vi "DimostratoreTest.vi"() -> ()   [LabVIEW 2019]
doc: "Dimostratore API\n\nFunzionamento:\n1. Seleziona postazione e data\n Conferma\n Ottieni un array con tutti i test della postazione selezionata in base alla data\n2. Seleziona quale test eseguire\n Conferma che tutti gli assets dei test sono disponibili\n Mostra tutti gli step di un test\n3. Seleziona Step da eseguire inserendo anche un valore di prova\n Il risultato dello step viene riprodotto nell'outcome\n\nFunzionamento alternativo\n1. Imposta uno Step Id e conferma\n2. Inserisci un valore di prova e ottieni l'outcome"
uses:
  ByteGSAPIBase.lvclass
  TypeDef/MachineStates.ctl
  TypeDef/Test.ctl
  TypeDef/Asset.ctl
  TypeDef/Step.ctl
  <vilib>/Utility/miscctls.llb/LVStringsAndValuesArrayTypeDef_I32.ctl
panel:
  in  "Exit":bool=TRUE
  out "Step Name":string
  in  "Home":bool
  in  "Indietro":bool
  out "Infos":string
  in  "Duration":dbl
  in  "Ottieni Passaggio Step":bool
  in  "Step Id":i32
  in  "Valore Prova":dbl
  in  "Inizia Step":bool
  in  "Seleziona Step":i32(ring) items=["Plug and set the Power Supply"=36]
  in  "Inizia Test":bool
  in  "Seleziona Test":i32(ring)
  out "error out":errorcluster
  in  "error in (no error)":errorcluster
  in  "Ottieni Test Per Postazione":bool
  in  "ByteGSAPIBase in":refnum<class "ByteGSAPIBase.lvclass">
  in  "Data Partenza":timestamp format="%<%x>T"
  in  "Postazione":enum16{"POST 1", "POST 2"}(ring)
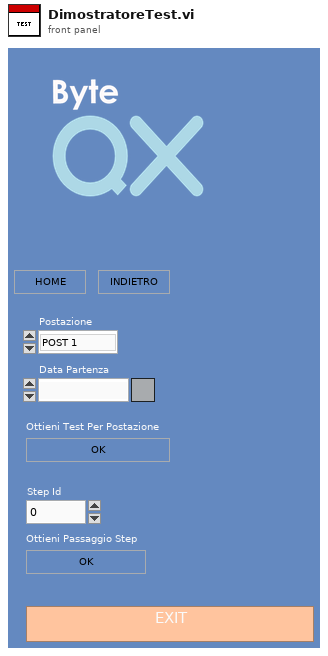
[diagram p1: front panel]
types:
  T1 = typedef "ByteGSWebAPI.lvlib/ByteGSAPIBase.lvclass/Step.ctl" = cluster{"id":i32, "descrizione":string, "prova":string, "assets":T2[], "criterio_accettazione":string, "valore_criterio_accettazione_max":dbl, "valore_criterio_accettazione_min":dbl, "udm_criterio_accettazione":string, "duration_prova":string, "udm_duration_prova":string, "valore_prova":dbl, "outcome":string, "ordine":i32, "user":i32, "link_automation":string, "instruction_automation":string, "data_completamento_checklist":timestamp}
  T2 = typedef "ByteGSWebAPI.lvlib/ByteGSAPIBase.lvclass/Asset.ctl" = cluster{"descrizione":string, "slug":string, "id":i32}
  T3 = typedef "ByteGSWebAPI.lvlib/ByteGSAPIBase.lvclass/Test.ctl" = cluster{"titolo":string, "descrizione":string, "statoprova":string, "assets":T2[], "id":i32, "data_apertura_prova":timestamp}
  T4 = typedef "MachineStates.ctl" = enum16{"Initialize", "Idle", "GetLimsTestsForBench", "AssetsCheck", "GetLimsTestSteps", "UpdateLimsTestStep", "GetLimsTestStep", "Indietro", "UpdateLimsTestStepAutomation"}
  T5 = cluster{"Postazione":refnum<vi>, "Data Partenza":refnum<vi>, "Ottieni Test Per Postazione":refnum<vi>, "Step Id":refnum<vi>, "Ottieni Passaggio Step":refnum<vi>, "Seleziona Test":refnum<vi>, "Inizia Test":refnum<vi>, "Seleziona Step":refnum<vi>, "Valore Prova":refnum<vi>, "Inizia Step":refnum<vi>, "Infos":refnum<vi>, "Duration":refnum<vi>, "Step Name":refnum<vi>, "Exit":refnum<vi>}
  T6 = cluster{"ByteGSAPIBase in":refnum<class "ByteGSAPIBase.lvclass">, "Array dei Test":T3[], "Steps Array":T1[]}
  T7 = typedef "LVStringsAndValuesArrayTypeDef_I32.ctl" = cluster{"String":string, "Value":i32}[]
  T8 = cluster{"Postazione":enum16{"POST 1", "POST 2"}, "Data Partenza":timestamp, "Seleziona Test":i32, "Seleziona Step":i32, "Valore Prova":dbl, "Step Id":i32, "Duration":dbl}
  T9 = cluster{"Postazione":enum16{"POST 1", "POST 2"}, "Data Partenza":timestamp}
  T10 = typedef "UpdateLimsTestStepData.ctl" = cluster{"duration_prova":string, "udm_duration_prova":string, "valore_prova":dbl, "outcome":string, "data_completamento_checklist":timestamp, "link_automation":string, "instruction_automation":string}
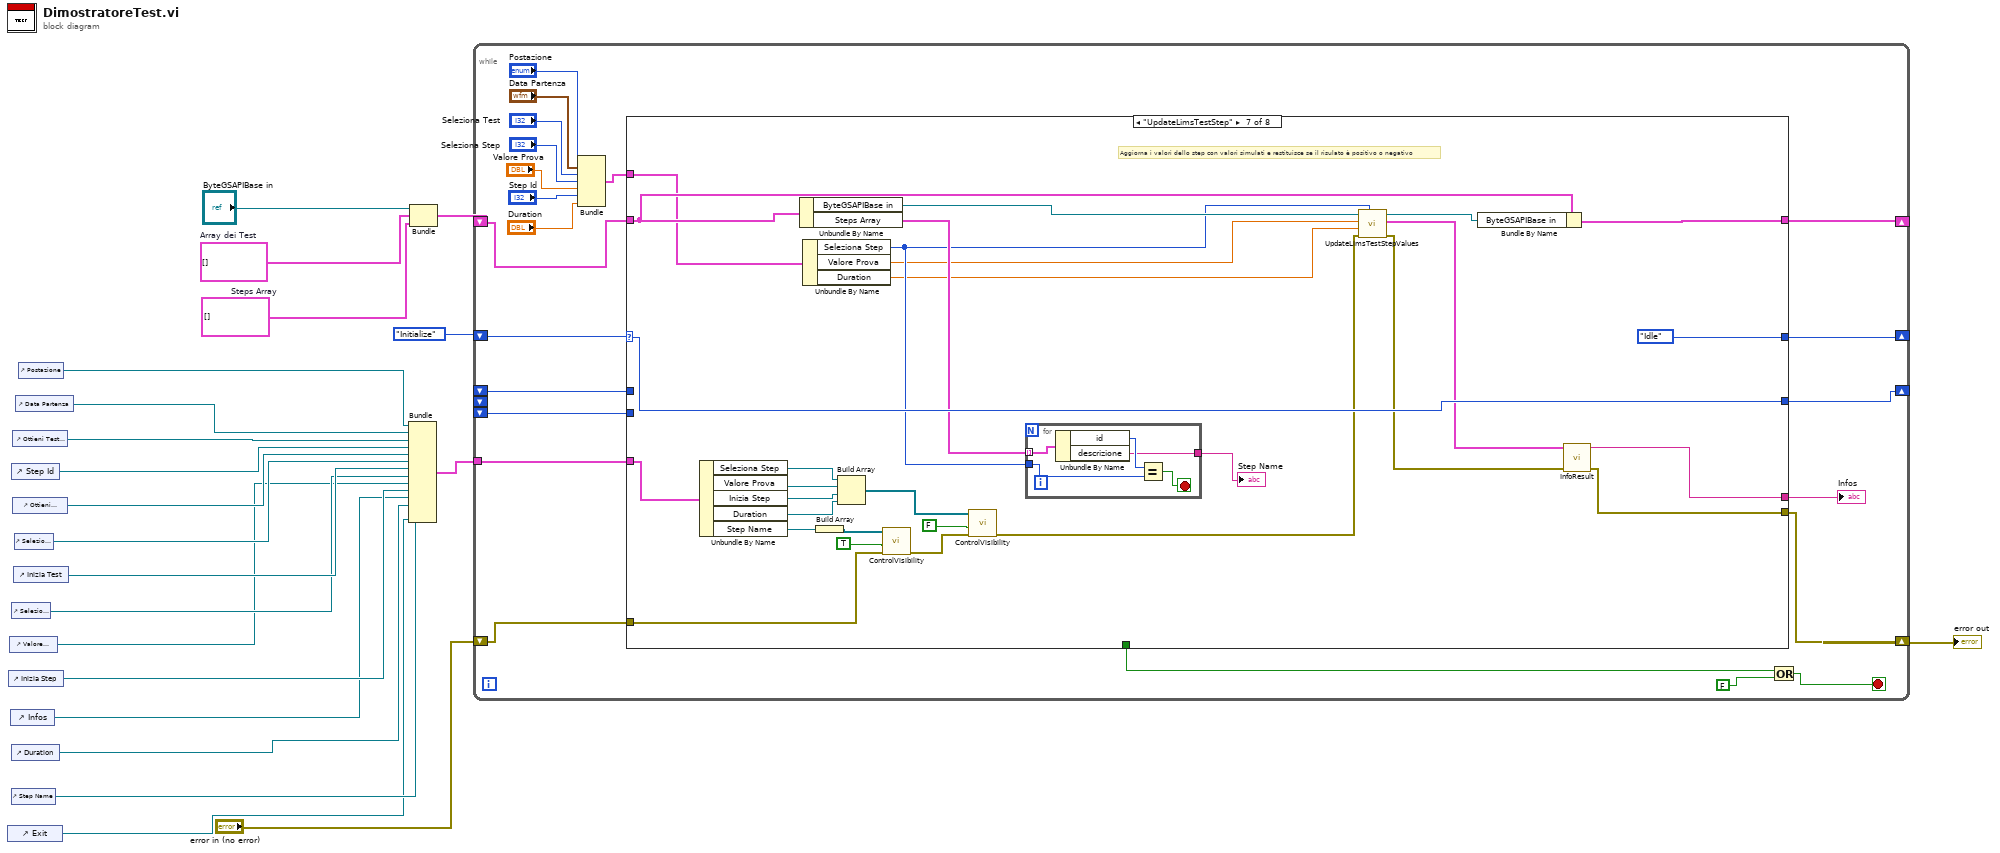
[diagram p0: block diagram]
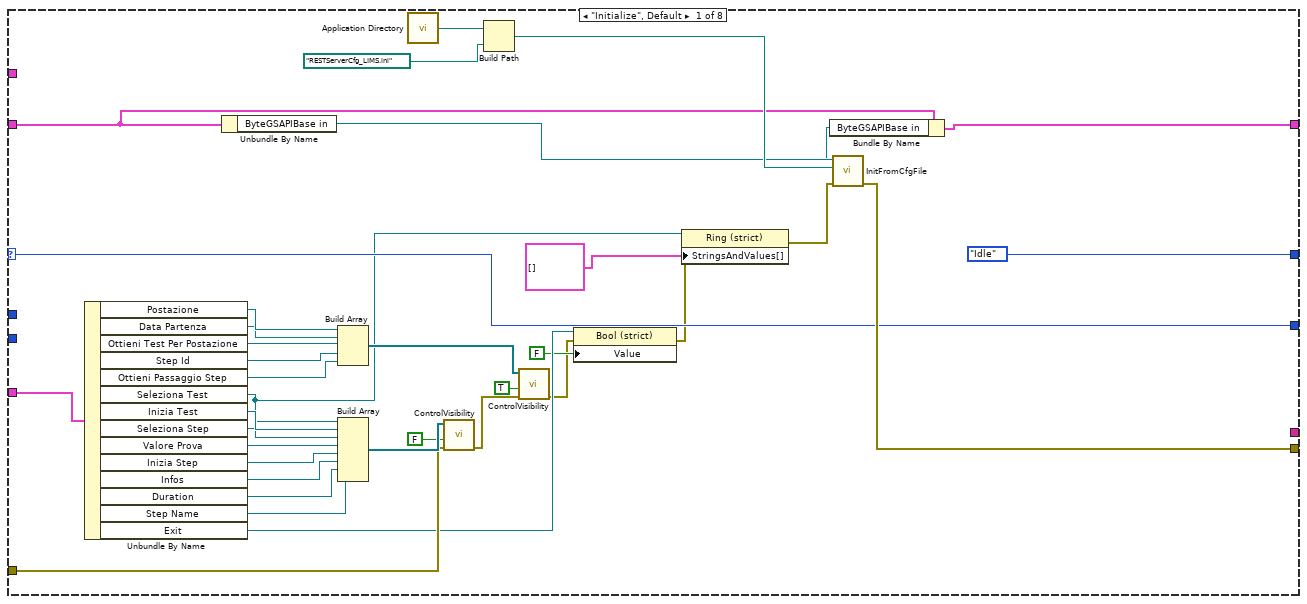
[diagram p2: hidden frame]
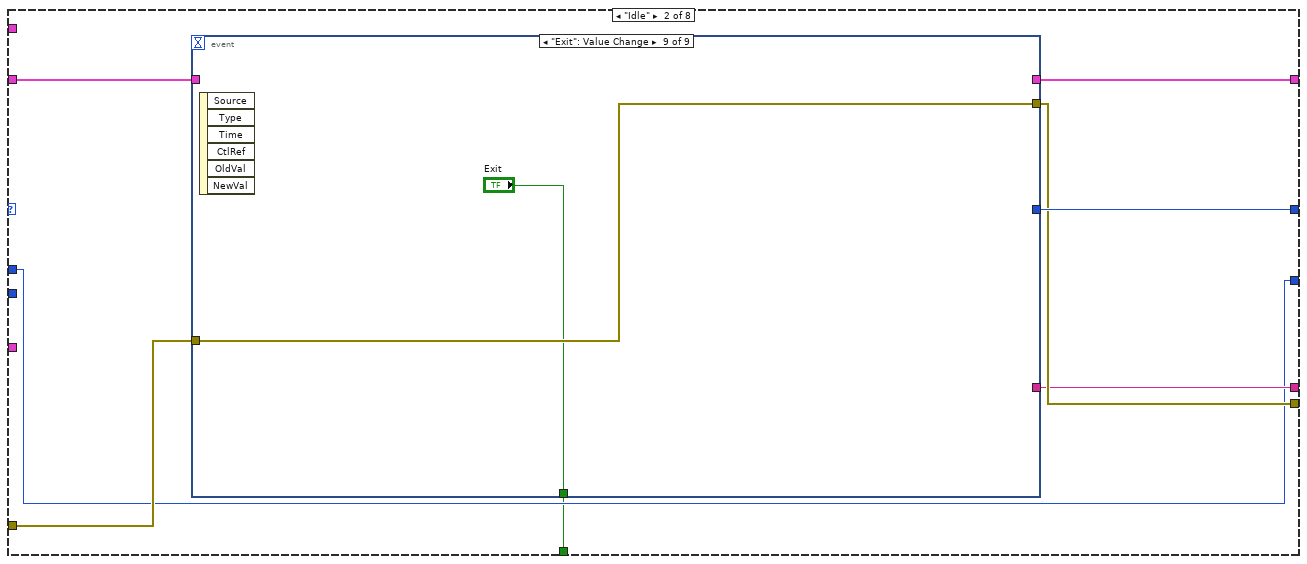
[diagram p3: hidden frame]
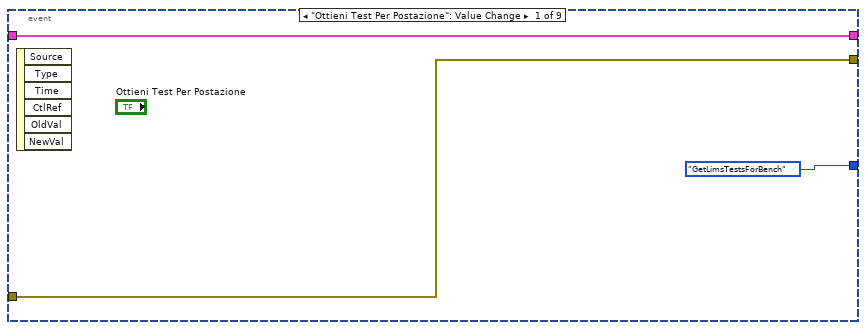
[diagram p4: hidden frame]
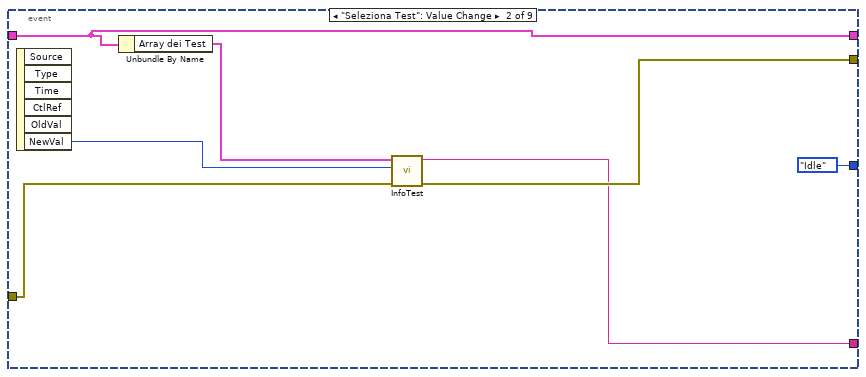
[diagram p5: hidden frame]
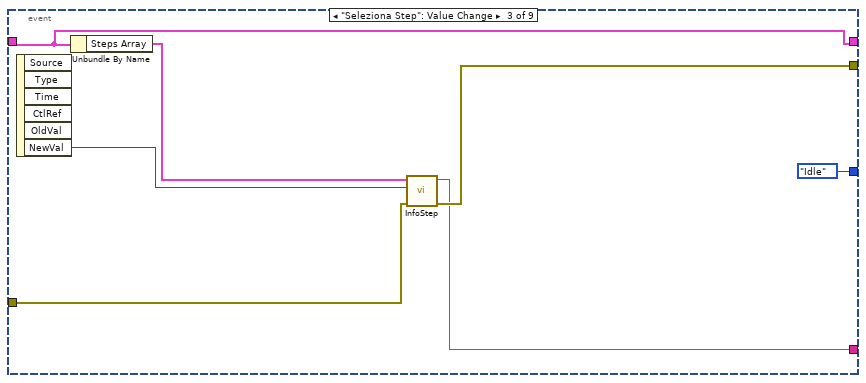
[diagram p6: hidden frame]
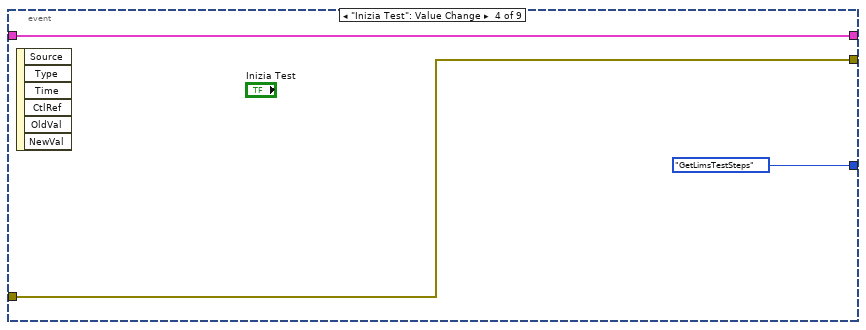
[diagram p7: hidden frame]
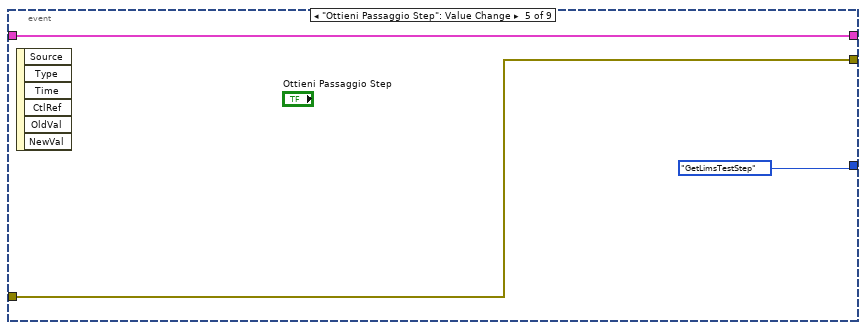
[diagram p8: hidden frame]
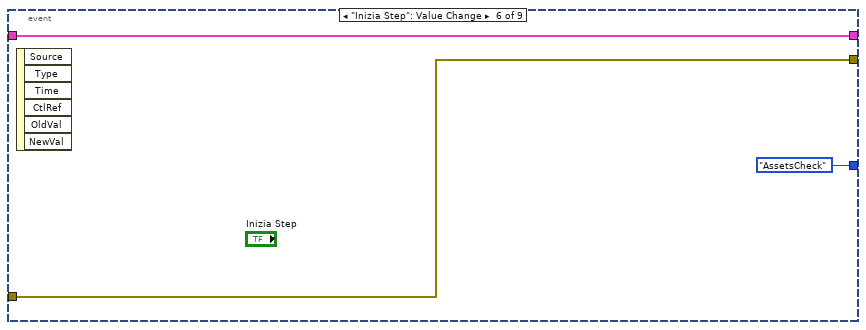
[diagram p9: hidden frame]
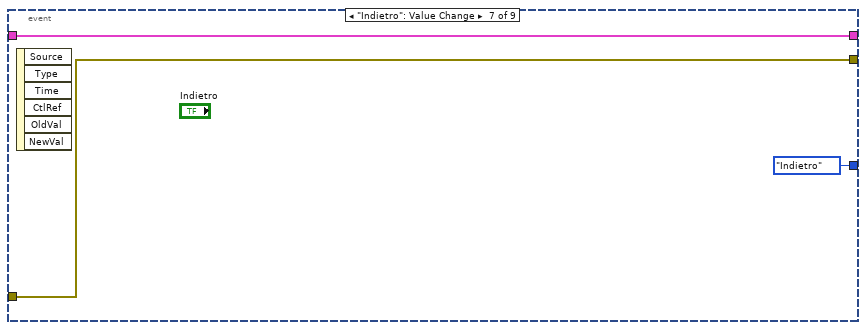
[diagram p10: hidden frame]
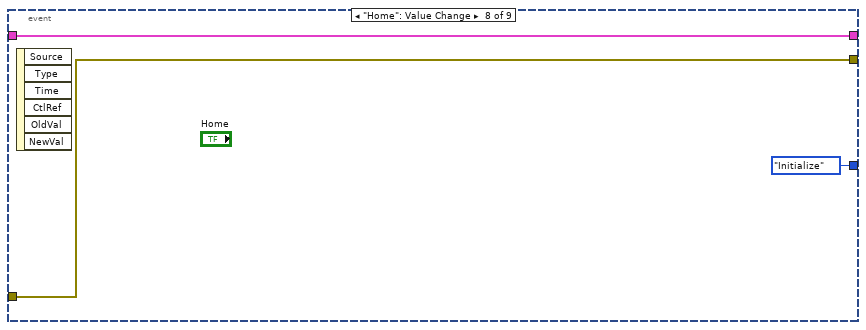
[diagram p11: hidden frame]
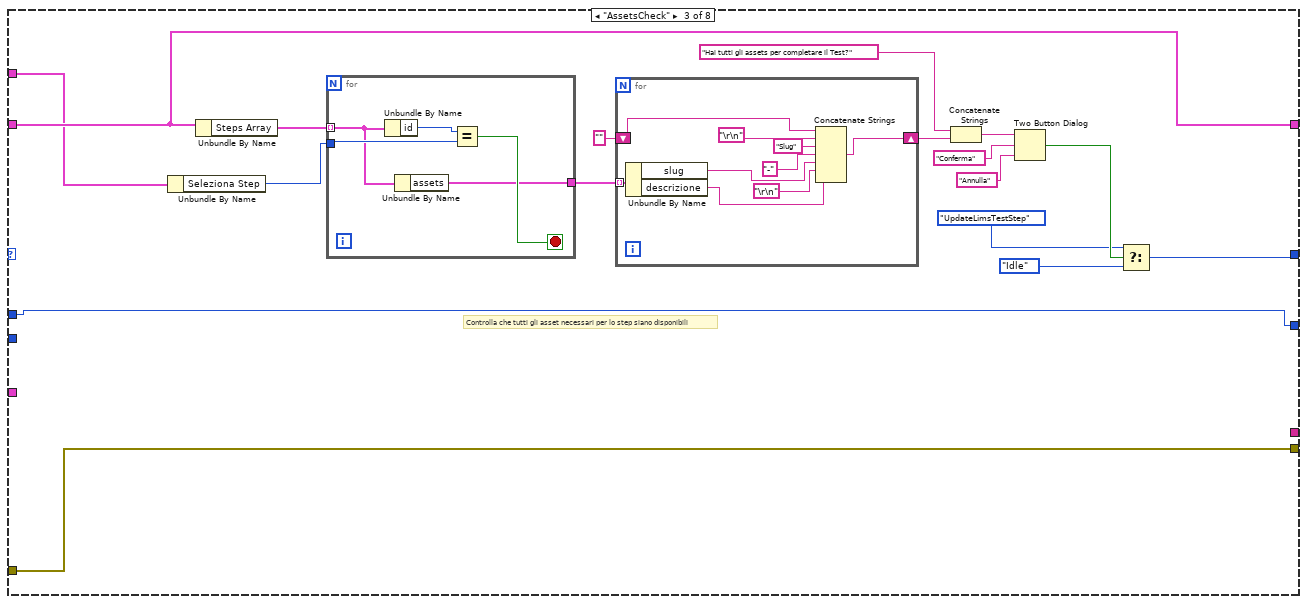
[diagram p12: hidden frame]
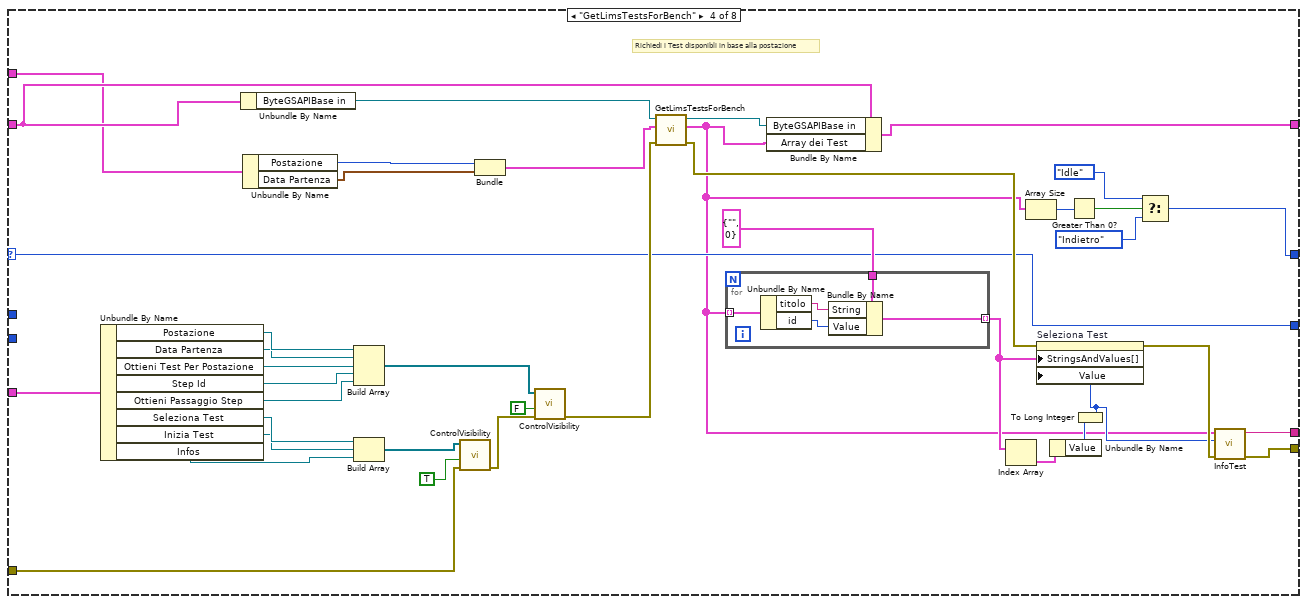
[diagram p13: hidden frame]
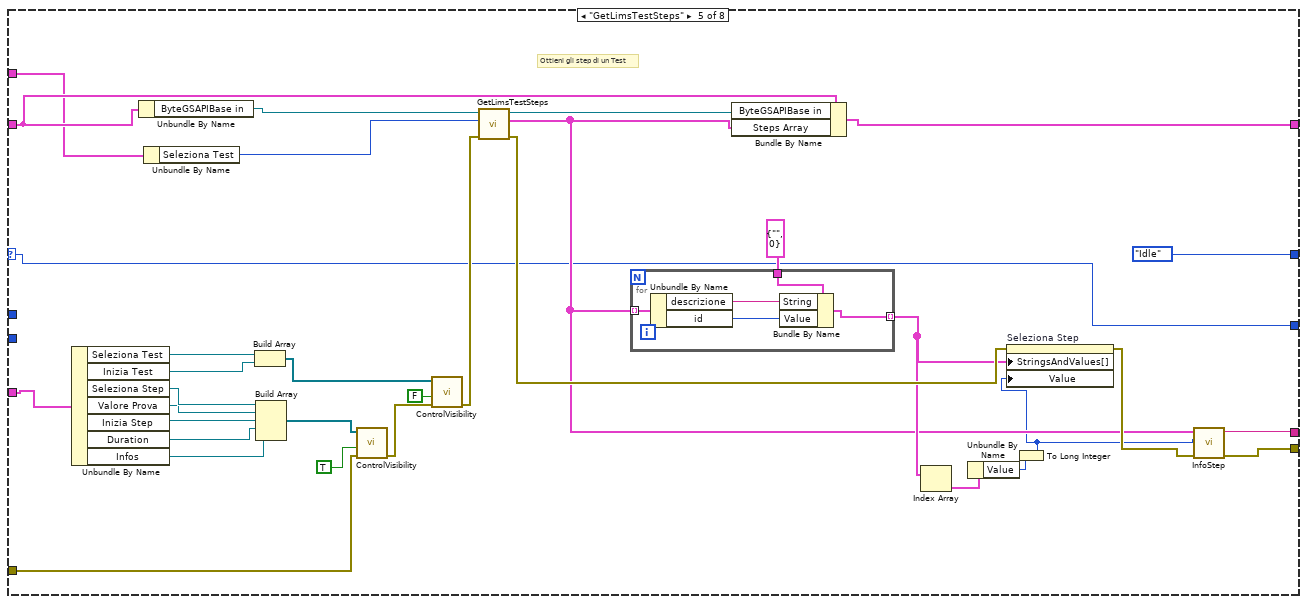
[diagram p14: hidden frame]
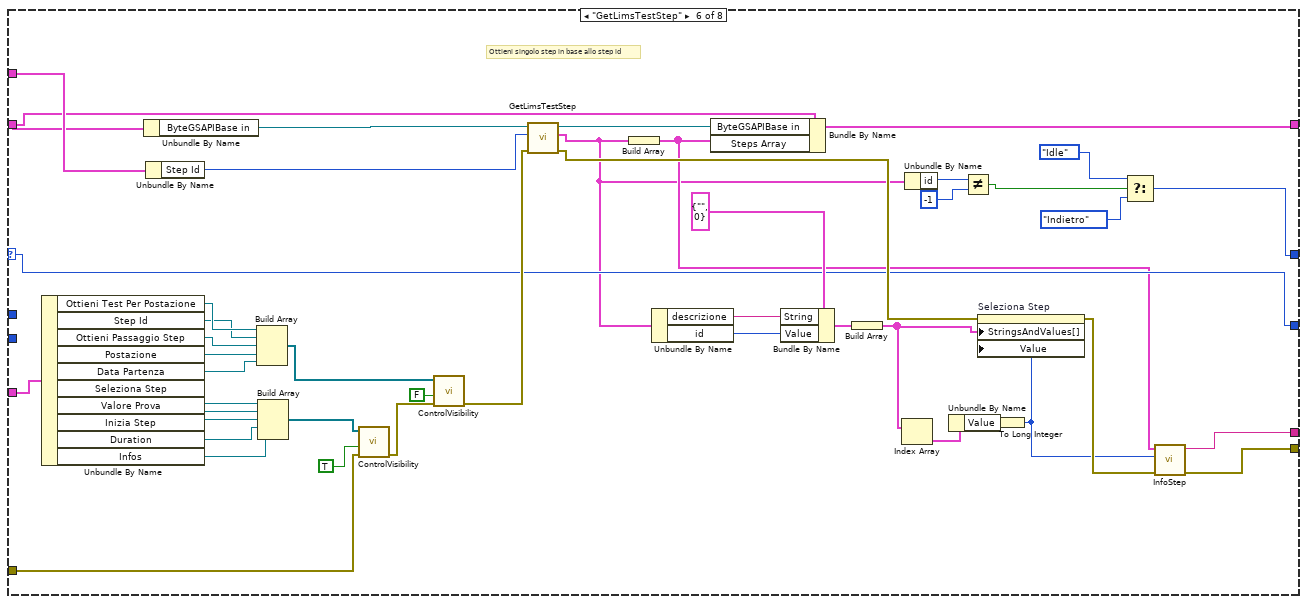
[diagram p15: hidden frame]
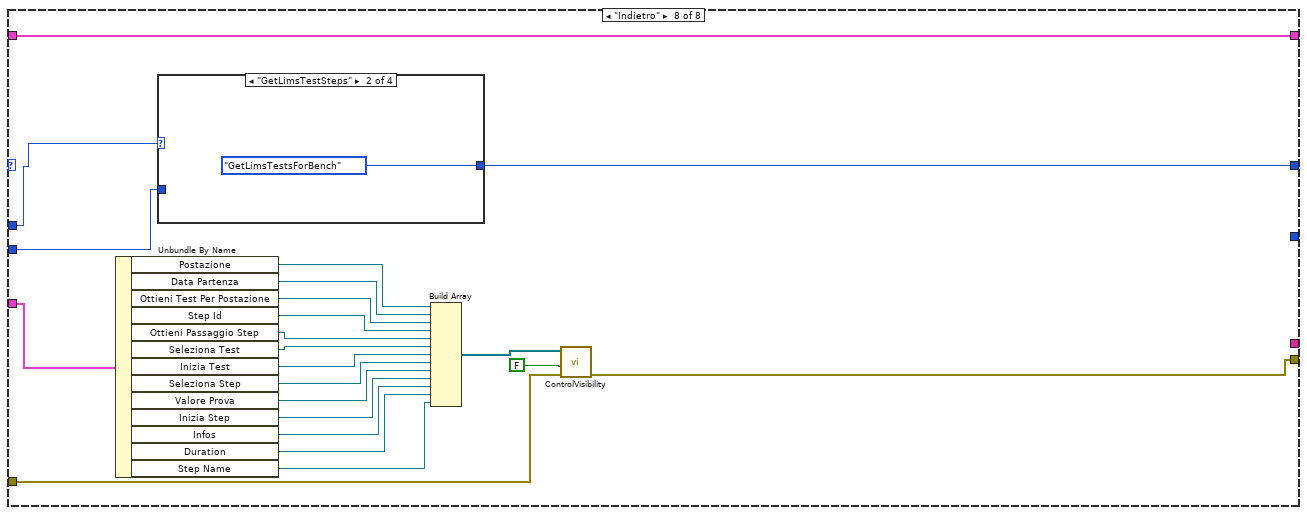
[diagram p16: hidden frame]
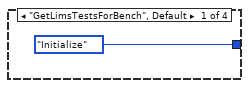
[diagram p17: hidden frame]
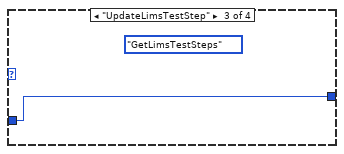
[diagram p18: hidden frame]
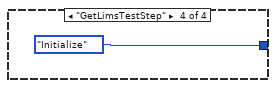
[diagram p19: hidden frame]
diagram:
  w19 = T1[] []  # Steps Array
  w21 = T3[] []  # Array dei Test
  n1 = control-ref of="Exit"() -> (w1:refnum<vi>)
  n2 = control-ref of="Inizia Step"() -> (w7:refnum<vi>)
  n3 = control-ref of="Valore Prova"() -> (w8:refnum<vi>)
  n4 = control-ref of="Infos"() -> (w3:refnum<vi>)
  n5 = control-ref of="Step Id"() -> (w13:refnum<vi>)
  n6 = control-ref of="Seleziona Step"() -> (w9:refnum<vi>)
  n7 = control-ref of="Duration"() -> (w5:refnum<vi>)
  n8 = control-ref of="Step Name"() -> (w2:refnum<vi>)
  n9 = control-ref of="Ottieni Test Per Postazione"() -> (w14:refnum<vi>)
  n10 = control-ref of="Ottieni Passaggio Step"() -> (w12:refnum<vi>)
  n11 = control-ref of="Inizia Test"() -> (w10:refnum<vi>)
  n12 = control-ref of="Seleziona Test"() -> (w11:refnum<vi>)
  n13 = control-ref of="Data Partenza"() -> (w15:refnum<vi>)
  n14 = control-ref of="Postazione"() -> (w16:refnum<vi>)
  n15 = Bundle("Postazione"=w16, "Data Partenza"=w15, "Ottieni Test Per Postazione"=w14, "Step Id"=w13, "Ottieni Passaggio Step"=w12, "Seleziona Test"=w11, "Inizia Test"=w10, "Seleziona Step"=w9, "Valore Prova"=w8, "Inizia Step"=w7, "Infos"=w3, "Duration"=w5, "Step Name"=w2, "Exit"=w1) -> (w6:T5)  [unwired: 1 in]
  n16 = Bundle("ByteGSAPIBase in"="ByteGSAPIBase in", "Array dei Test"=w21, "Steps Array"=w19) -> (w18:T6)  [unwired: 1 in]
  n17 = while {
    shift-right: [w43] -> _
    shift-left: MachineStates."Initialize" -> [w44]
    shift-right: [w42] -> _
    shift-left: w18 -> [w26]
    shift-right: [w40] -> w17
    shift-left: "error in (no error)" -> [w41]
    tunnel: w6 -> [w32]
    shift-right: [w30] -> _
    shift-left: _ -> [w29]
    shift-left: _ -> [_]
    shift-left: _ -> [w28]
    stop <- w24 stop-if-true
    n18 = Bundle("Postazione"="Postazione", "Data Partenza"="Data Partenza", "Seleziona Test"="Seleziona Test", "Seleziona Step"="Seleziona Step", "Valore Prova"="Valore Prova", "Step Id"="Step Id", "Duration"="Duration") -> (w34:T8)  [unwired: 1 in]
    n19 = case shown="\"UpdateLimsTestStep\"" w44 {
      selector: w44 -> [w53 _ _ w161 w201 w246 w304 _]
      tunnel: [MachineStates."Idle" w88 w130 w155 MachineStates."Idle" w242 MachineStates."Idle" w318] -> w43
      tunnel: w26 -> [w75 w87 w137 w193 w230 w277 w309 w337]
      tunnel: [w73 w86 w137 w192 w228 w278 w307 w337] -> w42
      tunnel: w41 -> [w56 w85 w139 w162 w208 w253 w286 w321]
      tunnel: [w72 w84 w139 w179 w206 w250 w301 w320] -> w40
      tunnel: w34 -> [_ _ w126 w188 w222 w281 w305 _]
      tunnel: w32 -> [w71 _ _ w165 w217 w257 w298 w327]
      tunnel: [_ w83 _ w178 w207 w249 w300 _] -> w27
      tunnel: [w53 w82 w123 w161 w201 w246 w304 _] -> w30
      tunnel: w29 -> [_ w82 w123 _ _ _ _ w319]
      tunnel: w28 -> [_ _ _ _ _ _ _ w317]
      tunnel: [_ w81 _ _ _ _ _ _] -> w23
      frame "Initialize", Default {
        n20 = Unbundle By Name(w71) -> ("Postazione"=w65:refnum<vi>, "Data Partenza"=w64:refnum<vi>, "Ottieni Test Per Postazione"=w63:refnum<vi>, "Step Id"=w62:refnum<vi>, "Ottieni Passaggio Step"=w61:refnum<vi>, "Seleziona Test"=w51:refnum<vi>, "Inizia Test"=w70:refnum<vi>, "Seleziona Step"=w69:refnum<vi>, "Valore Prova"=w68:refnum<vi>, "Inizia Step"=w67:refnum<vi>, "Infos"=w66:refnum<vi>, "Duration"=w54:refnum<vi>, "Step Name"=w52:refnum<vi>, "Exit"=w48:refnum<vi>)
        n21 = Unbundle By Name(w75) -> ("ByteGSAPIBase in"=w76:refnum<class "ByteGSAPIBase.lvclass">)
        n22 = Build Array(w65, w64, w63, w62, w61) -> (w59:refnum<vi>[])
        n23 = Build Array(w51, w70, w69, w68, w67, w66, w54, w52) -> (w60:refnum<vi>[])
        n24 = call <vilib>:"Application Directory.vi"() -> ("Application Directory"=w78:path)
        n25 = call "ControlVisibility.vi"("error in (no error)"=w56, "Visible"=FALSE, "Controls"=w60) -> ("error out"=w55:errorcluster)  [unwired: 8 in]
        n26 = Build Path(base path=w78, name or relative path=path "RESTServerCfg_LIMS.ini") -> (appended path=w79:path)
        n27 = call "ControlVisibility.vi"("error in (no error)"=w55, "Visible"=TRUE, "Controls"=w59) -> ("error out"=w45:errorcluster)  [unwired: 8 in]
        n28 = property class="Bool (strict)"(reference=w48, error in=w45, "Value"=FALSE) -> (error out=w46:errorcluster)  [unwired: 1 out]
        n29 = property class="Ring (strict)"(reference=w51, error in=w46, "StringsAndValues[]"=T7 [] ("Strings And Values []")) -> (error out=w50:errorcluster)  [unwired: 1 out]
        n30 = call-dynamic "InitFromCfgFile.vi"("error in (no error)"=w50, "configuration file path"=w79, "ByteGSAPIBase in"=w76) -> ("error out"=w72:errorcluster, "ByteGSAPIBase out"=w74:refnum<class "ByteGSAPIBase.lvclass">)  [unwired: 7 in]
        n31 = Bundle By Name(cluster=w75, "ByteGSAPIBase in"=w74) -> (w73:T6)
      }
      frame "Idle" {
        n32 = event shown="[8] \"Exit\": Value Change" {
          selector: _ -> [_ _ _ _ _ _ _ _ _]
          dyn-events: _ -> [_ _ _ _ _ _ _ _ _]
          timeout: _ -> [_ _ _ _ _ _ _ _ _]
          tunnel: [MachineStates."GetLimsTestsForBench" MachineStates."Idle" MachineStates."Idle" MachineStates."GetLimsTestSteps" MachineStates."GetLimsTestStep" MachineStates."AssetsCheck" MachineStates."Indietro" MachineStates."Initialize" _] -> w88
          tunnel: w87 -> [w89 w98 w104 w107 w111 w114 w116 w119 _]
          tunnel: [w89 w98 w104 w107 w111 w114 w116 w119 _] -> w86
          tunnel: w85 -> [w90 w97 w100 w106 w110 w113 w117 w120 w122]
          tunnel: [w90 w96 w102 w106 w110 w113 w117 w120 w122] -> w84
          tunnel: [_ w94 w101 _ _ _ _ _ _] -> w83
          tunnel: [_ _ _ _ _ _ _ _ "Exit"] -> w81
          event "Ottieni Test Per Postazione": Value Change {
            n33 = event-data() -> ()  [unwired: 1 in, 6 out]
          }
          event "Seleziona Test": Value Change {
            n34 = event-data() -> ("NewVal"=w92:i32)  [unwired: 1 in, 5 out]
            n35 = Unbundle By Name(w98) -> ("Array dei Test"=w93:T3[])
            n36 = call "InfoTest.vi"("error in"=w97, "Seleziona Test"=w92, "TestForBenchArray"=w93) -> ("error out"=w96:errorcluster, "Info Test"=w94:string)  [unwired: 7 in]
          }
          event "Seleziona Step": Value Change {
            n37 = event-data() -> ("NewVal"=w99:i32)  [unwired: 1 in, 5 out]
            n38 = Unbundle By Name(w104) -> ("Steps Array"=w105:T1[])
            n39 = call "InfoStep.vi"("error in"=w100, "Seleziona Step"=w99, "Test Steps List"=w105) -> ("error out"=w102:errorcluster, "Info Test"=w101:string)  [unwired: 7 in]
          }
          event "Inizia Test": Value Change {
            n40 = event-data() -> ()  [unwired: 1 in, 6 out]
          }
          event "Ottieni Passaggio Step": Value Change {
            n41 = event-data() -> ()  [unwired: 1 in, 6 out]
          }
          event "Inizia Step": Value Change {
            n42 = event-data() -> ()  [unwired: 1 in, 6 out]
          }
          event "Indietro": Value Change {
            n43 = event-data() -> ()  [unwired: 1 in, 6 out]
          }
          event "Home": Value Change {
            n44 = event-data() -> ()  [unwired: 1 in, 6 out]
          }
          event "Exit": Value Change {
            n45 = event-data() -> ()  [unwired: 1 in, 6 out]
          }
        }
      }
      frame "AssetsCheck" {
        # "Controlla che tutti gli asset necessari per lo step siano disponibili"
        n46 = Unbundle By Name(w126) -> ("Seleziona Step"=w125:i32)
        n47 = Unbundle By Name(w137) -> ("Steps Array"=w138:T1[])
        n48 = for {
          tunnel: w138 -> [w150] mode=indexing
          tunnel: w125 -> [w152]
          tunnel: [w149] -> w136
          stop <- w151 stop-if-true
          n49 = Unbundle By Name(w150) -> ("id"=w153:i32)
          n50 = Unbundle By Name(w150) -> ("assets"=w149:T2[])
          n51 = Equal?(x=w153, y=w152) -> (x = y?=w151:bool)
        }
        n52 = for {
          tunnel: w136 -> [w147] mode=indexing
          shift-right: [w148] -> w135
          shift-left: "" -> [w146]
          n53 = Unbundle By Name(w147) -> ("slug"=w140:string, "descrizione"=w141:string)
          n54 = Concatenate Strings(w146, "\r\n", "Slug" ("string"), "-", w140, "\r\n", w141) -> (w148:string)
        }
        n55 = Concatenate Strings("Hai tutti gli assets per completare il Test?", w135) -> (w133:string)
        n56 = Two Button Dialog(message=w133, 1:"Annulla" ("F button name (\"Cancel\")"), 2:"Conferma" ("T button name (\"OK\")")) -> (T button?=w129:bool)
        n57 = Select(t=MachineStates."UpdateLimsTestStep", s=w129, f=MachineStates."Idle") -> (s? t:f=w130:T4)
      }
      frame "GetLimsTestsForBench" {
        # "Richiedi i Test disponibli in base alla postazione"
        n58 = Unbundle By Name(w165) -> ("Postazione"=w175:refnum<vi>, "Data Partenza"=w174:refnum<vi>, "Ottieni Test Per Postazione"=w173:refnum<vi>, "Step Id"=w172:refnum<vi>, "Ottieni Passaggio Step"=w171:refnum<vi>, "Seleziona Test"=w177:refnum<vi>, "Inizia Test"=w176:refnum<vi>, "Infos"=w164:refnum<vi>)
        n59 = Unbundle By Name(w193) -> ("ByteGSAPIBase in"=w185:refnum<class "ByteGSAPIBase.lvclass">)
        n60 = Unbundle By Name(w188) -> ("Postazione"=w187:enum16{"POST 1", "POST 2"}, "Data Partenza"=w186:timestamp)
        n61 = Build Array(w175, w174, w173, w172, w171) -> (w169:refnum<vi>[])
        n62 = Build Array(w177, w176, w164) -> (w170:refnum<vi>[])
        n63 = call "ControlVisibility.vi"("error in (no error)"=w162, "Visible"=TRUE, "Controls"=w170) -> ("error out"=w166:errorcluster)  [unwired: 8 in]
        n64 = Bundle("Postazione"=w187, "Data Partenza"=w186) -> (w182:T9)  [unwired: 1 in]
        n65 = call "ControlVisibility.vi"("error in (no error)"=w166, "Visible"=FALSE, "Controls"=w169) -> ("error out"=w163:errorcluster)  [unwired: 8 in]
        n66 = call-dynamic "GetLimsTestsForBench.vi"("error in (no error)"=w163, "Data in"=w182, "ByteGSAPIBase in"=w185) -> ("error out"=w184:errorcluster, "Tests for bench"=w159:T3[], "ByteGSAPIBase out"=w183:refnum<class "ByteGSAPIBase.lvclass">)  [unwired: 6 in]
        n67 = for {
          tunnel: w159 -> [w198] mode=indexing
          tunnel: [w195] -> w190 mode=indexing
          tunnel: cluster{"String":string, "Value":u16} {"String"="", "Value"=0} ("Cluster") -> [w194]
          n68 = Unbundle By Name(w198) -> ("titolo"=w197:string, "id"=w196:i32)
          n69 = Bundle By Name(cluster=w194, "String"=w197, "Value"=w196) -> (w195:cluster{"String":string, "Value":u16})
        }
        n70 = Bundle By Name(cluster=w193, "ByteGSAPIBase in"=w183, "Array dei Test"=w159) -> (w192:T6)
        n71 = Index Array(array=w190) -> (element=w189:cluster{"String":string, "Value":u16})  [unwired: 1 in]
        n72 = Array Size(array=w159) -> (size(s)=w158:i32)
        n73 = Unbundle By Name(w189) -> ("Value"=w181:u16)
        n74 = Greater Than 0?(x=w158) -> (x > 0?=w157:bool)
        n75 = To Long Integer(number=w181) -> (32bit integer=w160:i32)
        n76 = property on="Seleziona Test" class="Ring (strict)"(error in=w184, "StringsAndValues[]"=w190, "Value"=w160) -> (error out=w180:errorcluster)  [unwired: 1 in, 1 out]
        n77 = Select(t=MachineStates."Idle", s=w157, f=MachineStates."Indietro") -> (s? t:f=w155:T4)
        n78 = call "InfoTest.vi"("error in"=w180, "Seleziona Test"=w160, "TestForBenchArray"=w159) -> ("error out"=w179:errorcluster, "Info Test"=w178:string)  [unwired: 7 in]
      }
      frame "GetLimsTestSteps" {
        # "Ottieni gli step di un Test"
        n79 = Unbundle By Name(w217) -> ("Seleziona Test"=w216:refnum<vi>, "Inizia Test"=w215:refnum<vi>, "Seleziona Step"=w214:refnum<vi>, "Valore Prova"=w213:refnum<vi>, "Inizia Step"=w212:refnum<vi>, "Duration"=w202:refnum<vi>, "Infos"=w200:refnum<vi>)
        n80 = Unbundle By Name(w230) -> ("ByteGSAPIBase in"=w231:refnum<class "ByteGSAPIBase.lvclass">)
        n81 = Unbundle By Name(w222) -> ("Seleziona Test"=w221:i32)
        n82 = Build Array(w216, w215) -> (w211:refnum<vi>[])
        n83 = Build Array(w214, w213, w212, w202, w200) -> (w210:refnum<vi>[])
        n84 = call "ControlVisibility.vi"("error in (no error)"=w208, "Visible"=TRUE, "Controls"=w210) -> ("error out"=w218:errorcluster)  [unwired: 8 in]
        n85 = call "ControlVisibility.vi"("error in (no error)"=w218, "Visible"=FALSE, "Controls"=w211) -> ("error out"=w209:errorcluster)  [unwired: 8 in]
        n86 = call-dynamic "GetLimsTestSteps.vi"("error in (no error)"=w209, "Test-id"=w221, "ByteGSAPIBase in"=w231) -> ("error out"=w225:errorcluster, "Test Steps List"=w203:T1[], "ByteGSAPIBase out"=w229:refnum<class "ByteGSAPIBase.lvclass">)  [unwired: 6 in]
        n87 = for {
          tunnel: w203 -> [w236] mode=indexing
          tunnel: [w235] -> w223 mode=indexing
          tunnel: cluster{"String":string, "Value":u16} {"String"="", "Value"=0} ("Cluster") -> [w234]
          n88 = Unbundle By Name(w236) -> ("descrizione"=w233:string, "id"=w232:i32)
          n89 = Bundle By Name(cluster=w234, "String"=w233, "Value"=w232) -> (w235:cluster{"String":string, "Value":u16})
        }
        n90 = Bundle By Name(cluster=w230, "ByteGSAPIBase in"=w229, "Steps Array"=w203) -> (w228:T6)
        n91 = Index Array(array=w223) -> (element=w224:cluster{"String":string, "Value":u16})  [unwired: 1 in]
        n92 = Unbundle By Name(w224) -> ("Value"=w205:u16)
        n93 = To Long Integer(number=w205) -> (32bit integer=w199:i32)
        n94 = property on="Seleziona Step" class="Ring (strict)"(error in=w225, "StringsAndValues[]"=w223, "Value"=w199) -> (error out=w204:errorcluster)  [unwired: 1 in, 1 out]
        n95 = call "InfoStep.vi"("error in"=w204, "Seleziona Step"=w199, "Test Steps List"=w203) -> ("error out"=w206:errorcluster, "Info Test"=w207:string)  [unwired: 7 in]
      }
      frame "GetLimsTestStep" {
        # "Ottieni singolo step in base allo step id"
        n96 = Unbundle By Name(w257) -> ("Ottieni Test Per Postazione"=w256:refnum<vi>, "Step Id"=w255:refnum<vi>, "Ottieni Passaggio Step"=w254:refnum<vi>, "Postazione"=w265:refnum<vi>, "Data Partenza"=w264:refnum<vi>, "Seleziona Step"=w263:refnum<vi>, "Valore Prova"=w262:refnum<vi>, "Inizia Step"=w261:refnum<vi>, "Duration"=w258:refnum<vi>, "Infos"=w247:refnum<vi>)
        n97 = Unbundle By Name(w277) -> ("ByteGSAPIBase in"=w280:refnum<class "ByteGSAPIBase.lvclass">)
        n98 = Unbundle By Name(w281) -> ("Step Id"=w279:i32)
        n99 = Build Array(w256, w255, w254, w265, w264) -> (w260:refnum<vi>[])
        n100 = Build Array(w263, w262, w261, w258, w247) -> (w259:refnum<vi>[])
        n101 = call "ControlVisibility.vi"("error in (no error)"=w253, "Visible"=TRUE, "Controls"=w259) -> ("error out"=w266:errorcluster)  [unwired: 8 in]
        n102 = call "ControlVisibility.vi"("error in (no error)"=w266, "Visible"=FALSE, "Controls"=w260) -> ("error out"=w252:errorcluster)  [unwired: 8 in]
        n103 = call-dynamic "GetLimsTestStep.vi"("error in (no error)"=w252, "Step-id"=w279, "ByteGSAPIBase in"=w280) -> ("error out"=w269:errorcluster, "StepList"=w240:T1, "ByteGSAPIBase out"=w276:refnum<class "ByteGSAPIBase.lvclass">)  [unwired: 6 in]
        n104 = Build Array(w240) -> (w241:T1[])
        n105 = Unbundle By Name(w240) -> ("descrizione"=w273:string, "id"=w274:i32)
        n106 = Bundle By Name(cluster=w277, "ByteGSAPIBase in"=w276, "Steps Array"=w241) -> (w278:T6)
        n107 = Bundle By Name(cluster=cluster{"String":string, "Value":u16} {"String"="", "Value"=0} ("Cluster"), "String"=w273, "Value"=w274) -> (w271:cluster{"String":string, "Value":u16})
        n108 = Build Array(w271) -> (w270:cluster{"String":string, "Value":u16}[])
        n109 = Index Array(array=w270) -> (element=w275:cluster{"String":string, "Value":u16})  [unwired: 1 in]
        n110 = Unbundle By Name(w240) -> ("id"=w239:i32)
        n111 = Unbundle By Name(w275) -> ("Value"=w248:u16)
        n112 = Not Equal?(x=w239, y=-1) -> (x != y?=w237:bool)
        n113 = To Long Integer(number=w248) -> (32bit integer=w245:i32)
        n114 = property on="Seleziona Step" class="Ring (strict)"(error in=w269, "StringsAndValues[]"=w270, "Value"=w245) -> (error out=w251:errorcluster)  [unwired: 1 in, 1 out]
        n115 = Select(t=MachineStates."Idle", s=w237, f=MachineStates."Indietro") -> (s? t:f=w242:T4)
        n116 = call "InfoStep.vi"("error in"=w251, "Seleziona Step"=w245, "Test Steps List"=w241) -> ("error out"=w250:errorcluster, "Info Test"=w249:string)  [unwired: 7 in]
      }
      frame "UpdateLimsTestStep" {
        # "Aggiorna i valori dello step con valori simulati e restituisce se il risulato è positivo o negativo"
        n117 = Unbundle By Name(w298) -> ("Seleziona Step"=w296:refnum<vi>, "Valore Prova"=w295:refnum<vi>, "Inizia Step"=w294:refnum<vi>, "Duration"=w293:refnum<vi>, "Step Name"=w287:refnum<vi>)
        n118 = Unbundle By Name(w309) -> ("ByteGSAPIBase in"=w310:refnum<class "ByteGSAPIBase.lvclass">, "Steps Array"=w291:T1[])
        n119 = Unbundle By Name(w305) -> ("Seleziona Step"=w284:i32, "Valore Prova"=w283:dbl, "Duration"=w282:dbl)
        n120 = Build Array(w287) -> (w288:refnum<vi>[])
        n121 = Build Array(w296, w295, w294, w293) -> (w292:refnum<vi>[])
        n122 = call "ControlVisibility.vi"("error in (no error)"=w286, "Visible"=TRUE, "Controls"=w288) -> ("error out"=w285:errorcluster)  [unwired: 8 in]
        n123 = call "ControlVisibility.vi"("error in (no error)"=w285, "Visible"=FALSE, "Controls"=w292) -> ("error out"=w297:errorcluster)  [unwired: 8 in]
        n124 = for {
          tunnel: w284 -> [w314]
          tunnel: w291 -> [w315] mode=indexing
          tunnel: [w312] -> w290
          stop <- w311 stop-if-true
          n125 = Unbundle By Name(w315) -> ("id"=w313:i32, "descrizione"=w312:string)
          n126 = Equal?(x=w313, y=w314) -> (x = y?=w311:bool)
        }
        "Step Name" <- w290
        n127 = call-dynamic "UpdateLimsTestStepValues.vi"("step_id"=w284, "error in (no error)"=w297, "duration_hours"=w282, "value"=w283, "ByteGSAPIBase in"=w310) -> ("error out"=w302:errorcluster, "Result Step"=w303:T10, "ByteGSAPIBase out"=w308:refnum<class "ByteGSAPIBase.lvclass">)  [unwired: 4 in]
        n128 = Bundle By Name(cluster=w309, "ByteGSAPIBase in"=w308) -> (w307:T6)
        n129 = call "InfoResult.vi"("error in"=w302, "Result Step"=w303) -> ("error out"=w301:errorcluster, "Info Test"=w300:string)  [unwired: 8 in]
      }
      frame "Indietro" {
        n130 = Unbundle By Name(w327) -> ("Postazione"=w322:refnum<vi>, "Data Partenza"=w323:refnum<vi>, "Ottieni Test Per Postazione"=w324:refnum<vi>, "Step Id"=w325:refnum<vi>, "Ottieni Passaggio Step"=w326:refnum<vi>, "Seleziona Test"=w336:refnum<vi>, "Inizia Test"=w335:refnum<vi>, "Seleziona Step"=w334:refnum<vi>, "Valore Prova"=w333:refnum<vi>, "Inizia Step"=w332:refnum<vi>, "Infos"=w331:refnum<vi>, "Duration"=w328:refnum<vi>, "Step Name"=w316:refnum<vi>)
        n131 = case shown="\"GetLimsTestSteps\"" w319 {
          tunnel: [MachineStates."Initialize" MachineStates."GetLimsTestsForBench" w340 MachineStates."Initialize"] -> w318
          tunnel: w317 -> [_ _ w340 _]
          frame "GetLimsTestsForBench", Default {
          }
          frame "GetLimsTestSteps" {
          }
          frame "UpdateLimsTestStep" {
            (unwired) MachineStates."GetLimsTestSteps"
          }
          frame "GetLimsTestStep" {
          }
        }
        n132 = Build Array(w322, w323, w324, w325, w326, w336, w335, w334, w333, w332, w331, w328, w316) -> (w330:refnum<vi>[])
        n133 = call "ControlVisibility.vi"("error in (no error)"=w321, "Visible"=FALSE, "Controls"=w330) -> ("error out"=w320:errorcluster)  [unwired: 8 in]
      }
    }
    "Infos" <- w27
    n134 = Or(x=w23, y=FALSE) -> (x .or. y?=w24:bool)
  }
  "error out" <- w17
